vi "16portvalco_subVI_BM.vi"(8 "COM Port (16 Pos. Valve)":refnum<visa-resource-name>, 11 "Port Number":i32) -> (0 "error out":errorcluster)   [LabVIEW 2021]
uses:
  <vilib>/Instr/_visa.llb/VISA Configure Serial Port (Instr).vi
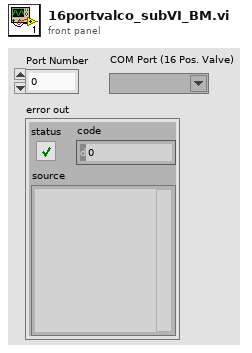
[diagram p1: front panel]
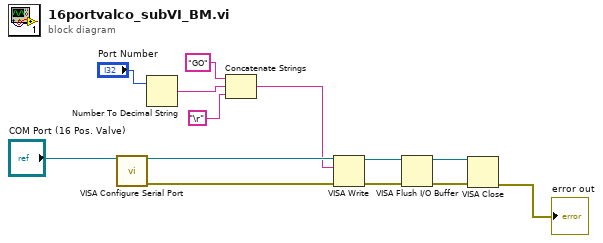
[diagram p0: block diagram]
diagram:
  n1 = call-poly "VISA Configure Serial Port"("VISA resource name"="COM Port (16 Pos. Valve)") -> ("VISA resource name out"=w8:refnum<visa-resource-name>, "error out"=w3:errorcluster)  [unwired: 13 in]
  n2 = Number To Decimal String(number="Port Number") -> (decimal integer string=w11:string)  [unwired: 1 in]
  n3 = Concatenate Strings("GO" ("string"), w11, "\r") -> (w1:string)
  n4 = VISA Write(VISA resource name=w8, write buffer=w1, error in (no error)=w3) -> (VISA resource name out=w7:refnum<visa-resource-name>, error out=w4:errorcluster)  [unwired: 1 out]
  n5 = VISA Flush I/O Buffer(VISA resource name=w7, error in (no error)=w4) -> (VISA resource name out=w6:refnum<visa-resource-name>, error out=w5:errorcluster)  [unwired: 1 in]
  n6 = VISA Close(VISA resource name=w6, error in (no error)=w5) -> (error out=→"error out":errorcluster)
